vi "FTW-CodeGen-GetTerms4.vi"(0 "State In":T2, 5 "XRef":refnum<vi>) -> (4 "Terms":T1(array[cluster]))   [LabVIEW 2013, in "FTW-SQLite-Insert.xnode"]
uses:
  FTW-SQLite-Insert.xnode
  FTW-CodeGen-State.ctl
panel:
  # "Inputs"
  # "Outputs"
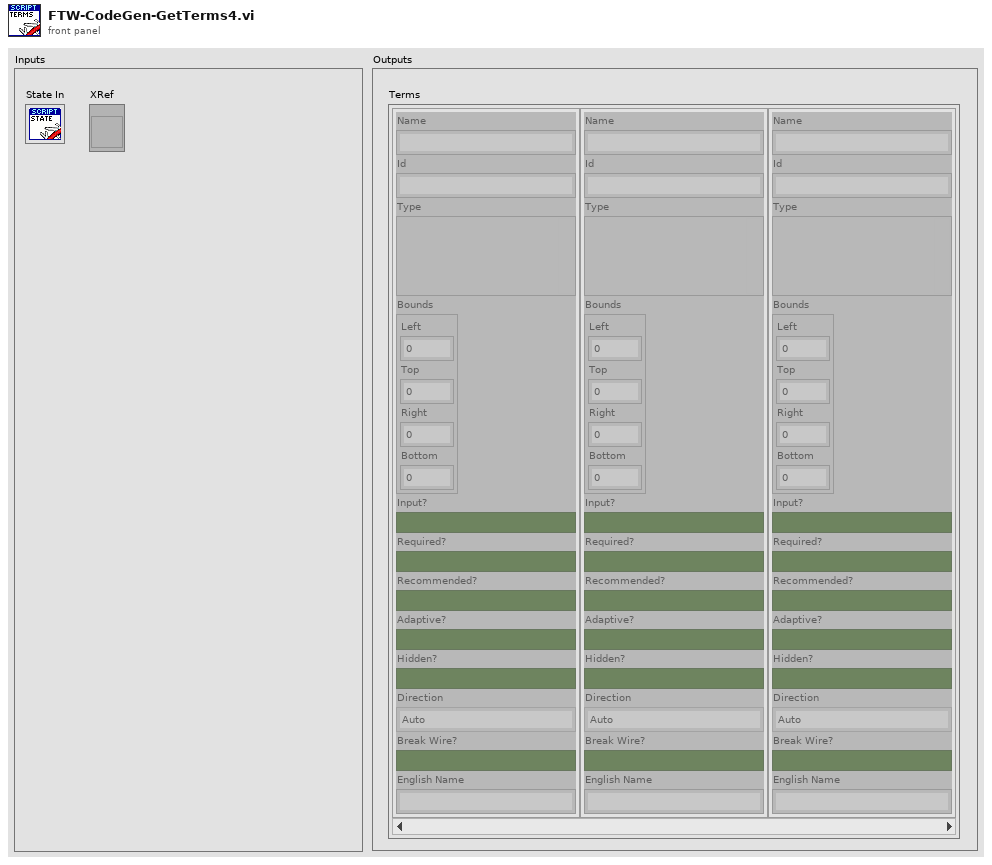
[diagram p1: front panel]
types:
  T1 = cluster{"Name":string, "Id":string, "Type":variant, "Bounds":cluster{"Left":i32, "Top":i32, "Right":i32, "Bottom":i32}, "Input?":bool, "Required?":bool, "Recommended?":bool, "Adaptive?":bool, "Hidden?":bool, "Direction":enum32{"Auto", "Up", "Down", "Left", "Right", "Center"}, "Break Wire?":bool, "English Name":string}[]
  T2 = typedef "FTW-SQLite-Insert.xnode/FTW-CodeGen-State.ctl" = cluster{"Dummy":string}
  T3 = cluster{"Name":string, "Id":string, "Type":variant, "Bounds":cluster{"Left":i32, "Top":i32, "Right":i32, "Bottom":i32}, "Input?":bool, "Required?":bool, "Recommended?":bool, "Adaptive?":bool, "Hidden?":bool, "Direction":enum32{"Auto", "Up", "Down", "Left", "Right", "Center"}, "Break Wire?":bool, "English Name":string}
  T4 = typedef "LVRectTypeDef.ctl" = cluster{"Left":i16, "Top":i16, "Right":i16, "Bottom":i16}
  T5 = enum16{"Invalid Wire Rule", "Required", "Recommended", "Optional", "Dynamic Dispatch"}[]
  T6 = enum16{"Invalid Wire Rule", "Required", "Recommended", "Optional", "Dynamic Dispatch"}
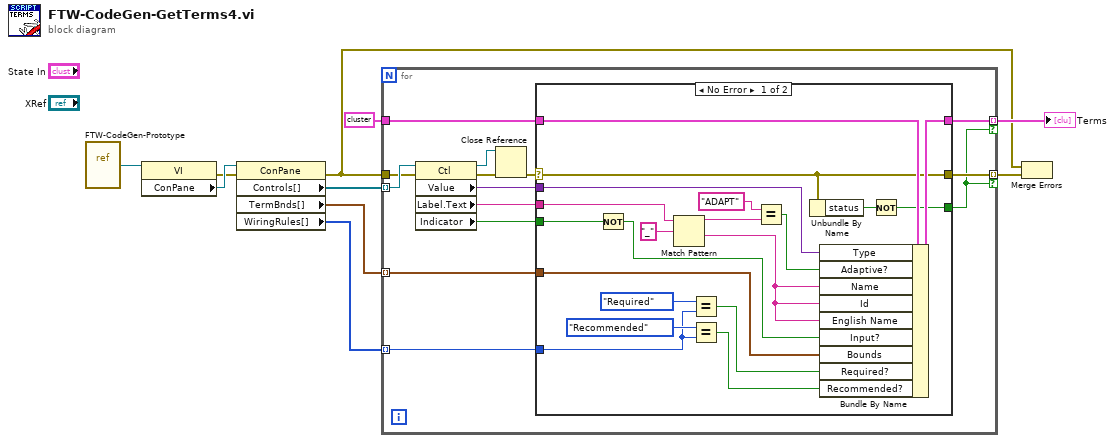
[diagram p0: block diagram]
diagram:
  n1 = vi-ref "FTW-CodeGen-Prototype.vi"() -> (w3:refnum<vi>)
  n2 = property class="VI"(reference=w3) -> (error out=w2:errorcluster, "ConPane"=w10:refnum<vi>)  [unwired: 1 in, 1 out]
  n3 = property class="ConPane"(reference=w10, error in=w2) -> (error out=w1:errorcluster, "Controls[]"=w9:refnum<vi>[], "TermBnds[]"=w6:T4[], "WiringRules[]"=w7:T5)  [unwired: 1 out]
  n4 = for {
    tunnel: w6 -> [w22] mode=indexing
    tunnel: w9 -> [w20] mode=indexing
    tunnel: w7 -> [w21] mode=indexing
    tunnel: T3 {"Name"="", "Id"="", "Type"=variant, "Bounds"={"Left"=0, "Top"=0, "Right"=0, "Bottom"=0}, "Input?"=FALSE, "Required?"=FALSE, "Recommended?"=FALSE, "Adaptive?"=FALSE, "Hidden?"=FALSE, "Direction"=enum."Auto", "Break Wire?"=FALSE, "English Name"=""} ("Term 4") -> [w24]
    tunnel: [w23] -> w4 mode=indexing if=w11
    tunnel: w1 -> [w16]
    tunnel: [w12] -> w5 mode=indexing if=w11
    n5 = property class="Ctl"(reference=w20, error in=w16) -> (reference out=w15:refnum<vi>, error out=w14:errorcluster, "Value"=w19:variant, "Label.Text"=w18:string, "Indicator"=w17:bool)
    n6 = Close Reference(reference=w15, error in (no error)=w14) -> (error out=w13:errorcluster)
    n7 = case shown="No Error" w13 {
      selector: w13 -> [w34 w45]
      tunnel: w24 -> [w44 w46]
      tunnel: [w43 w46] -> w23
      tunnel: w22 -> [w37 _]
      tunnel: w21 -> [w25 _]
      tunnel: w19 -> [w42 _]
      tunnel: w18 -> [w40 _]
      tunnel: w17 -> [w41 _]
      tunnel: [w33 _] -> w11
      tunnel: [w34 w45] -> w12
      frame No Error {
        n8 = Not(x=w41) -> (.not. x?=w36:bool)
        n9 = Match Pattern(string=w40, regular expression="_") -> (before substring=w32:string, after substring=w38:string)  [unwired: 1 in, 2 out]
        n10 = Equal?(x=T6."Required" ("Wire Rule"), y=w25) -> (x = y?=w27:bool)
        n11 = Equal?(x=T6."Recommended" ("Wire Rule"), y=w25) -> (x = y?=w26:bool)
        n12 = Equal?(x="ADAPT", y=w32) -> (x = y?=w30:bool)
        n13 = Unbundle By Name(w34) -> ("status"=w35:bool)
        n14 = Bundle By Name(cluster=w44, "Type"=w42, "Adaptive?"=w30, "Name"=w38, "Id"=w38, "English Name"=w38, "Input?"=w36, "Bounds"=w37, "Required?"=w27, "Recommended?"=w26) -> (w43:T3)
        n15 = Not(x=w35) -> (.not. x?=w33:bool)
      }
      frame Error {
      }
    }
  }
  "Terms" <- w4
  n16 = Merge Errors(w1, w5) -> ()  [unwired: 1 out]
